vi "Write SafetyLimits.vi"(8 "error in (no error)":errorcluster, 10 "SafetyLimits":T1, 11 "NhRegenGridSim in":refnum<class "NhRegenGridSim.lvclass">) -> (0 "error out":errorcluster, 3 "NhRegenGridSim out":refnum<class "NhRegenGridSim.lvclass">)   [LabVIEW 2018, in "AcPwrPlugins.lvlib" / "NhRegenGridSim.lvclass"]
uses:
  NhRegenGridSim.lvclass
  TypeDefs/SafetySettings.ctl
  NhRegenGridSim.lvclass/NhRegenGridSim.ctl
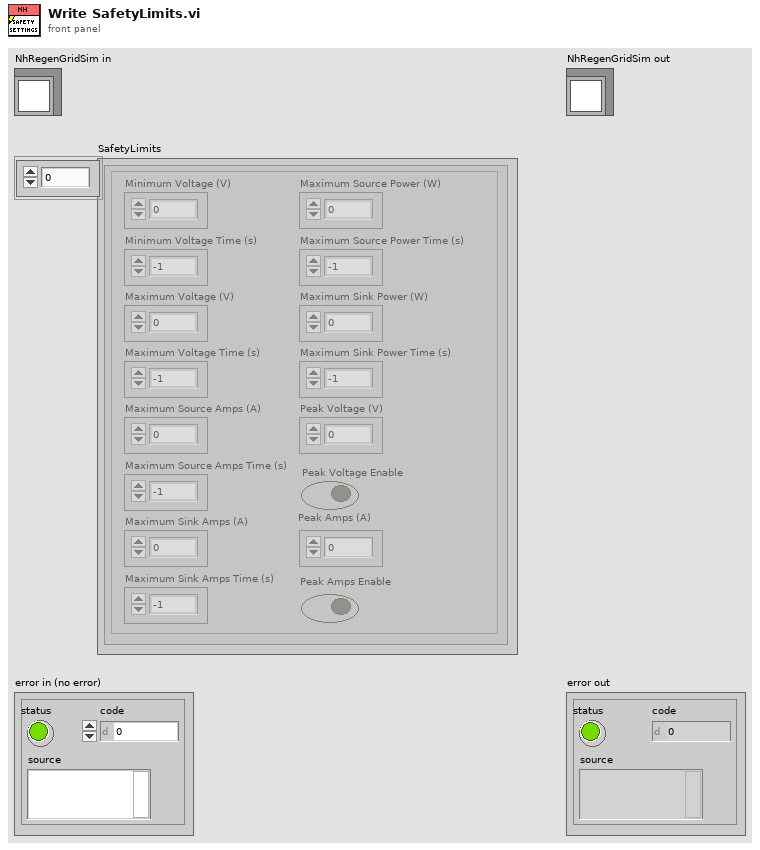
[diagram p1: front panel]
types:
  T1 = typedef "AcPwrPlugins.lvlib/NhRegenGridSim.lvclass/SafetySettings.ctl" = cluster{"Minimum Voltage (V)":dbl, "Minimum Voltage Time (s)":dbl, "Maximum Voltage (V)":dbl, "Maximum Voltage Time (s)":dbl, "Maximum Source Amps (A)":dbl, "Maximum Source Amps Time (s)":dbl, "Maximum Sink Amps (A)":dbl, "Maximum Sink Amps Time (s)":dbl, "Maximum Source Power (W)":dbl, "Maximum Source Power Time (s)":dbl, "Maximum Sink Power (W)":dbl, "Maximum Sink Power Time (s)":dbl, "Peak Voltage (V)":dbl, "Peak Voltage Enable":bool, "Peak Amps (A)":dbl, "Peak Amps Enable":bool}[]
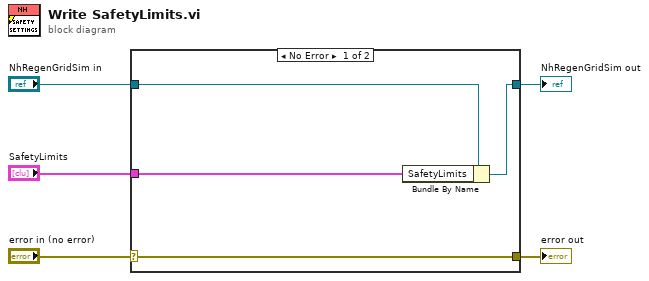
[diagram p0: block diagram]
diagram:
  n1 = case shown="No Error" "error in (no error)" {
    selector: "error in (no error)" -> [w9 w10]
    tunnel: [w9 w10] -> w4
    tunnel: [w7 w11] -> w2
    tunnel: "NhRegenGridSim in" -> [w8 w11]
    tunnel: "SafetyLimits" -> [w6 _]
    frame No Error {
      n2 = Bundle By Name(cluster=w8, "SafetyLimits"=w6) -> (w7:refnum<class "NhRegenGridSim.lvclass">)
    }
    frame Error {
    }
  }
  "error out" <- w4
  "NhRegenGridSim out" <- w2
